vi "Tokenizer Playground.vi"() -> ()   [LabVIEW 2019]
uses:
  Rectangle/Rectangle.lvclass
  ParsePaths/Path.lvclass
  Image/SVGImage.lvclass
  ParseXML/ParseSVG.lvclass
  Image/InitializationInfo.ctl
  ParseXML/ParseSVG.lvclass/ParseSVG.ctl
  Rectangle/InitializeInformation.ctl
panel:
  in  "string":string
  out "Image":refnum<class "SVGImage.lvclass">
  out "Paths":refnum<class "Path.lvclass">[](array[class])
  out "Rectangles":refnum<class "Rectangle.lvclass">[](array[class])
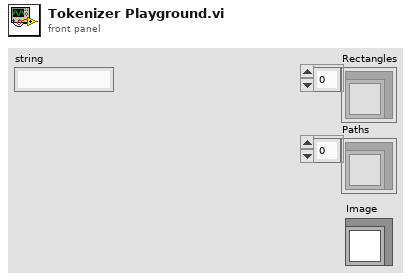
[diagram p1: front panel]
types:
  T1 = typedef "SVGImage.lvclass/InitializationInfo.ctl" = cluster{"X":string, "Y":string, "Width":string, "Height":string, "File Path":string, "ID":string}
  T2 = typedef "ParseSVG.lvclass/Path.ctl" = cluster{"d":string, "style":string, "transform":string, "id":string}
  T3 = typedef "ParseSVG.lvclass/Rect.ctl" = cluster{"style":string, "transform":string, "x":string, "y":string, "width":string, "height":string, "rx":string, "ry":string, "id":string}
  T4 = typedef "Rectangle.lvclass/InitializeInformation.ctl" = cluster{"X":string, "Y":string, "Width":string, "Height":string, "Rx":string, "Ry":string}
  T5 = typedef "ParseSVG.lvclass/Image.ctl" = cluster{"x":string, "y":string, "width":string, "height":string, "xlink:href":string, "id":string}
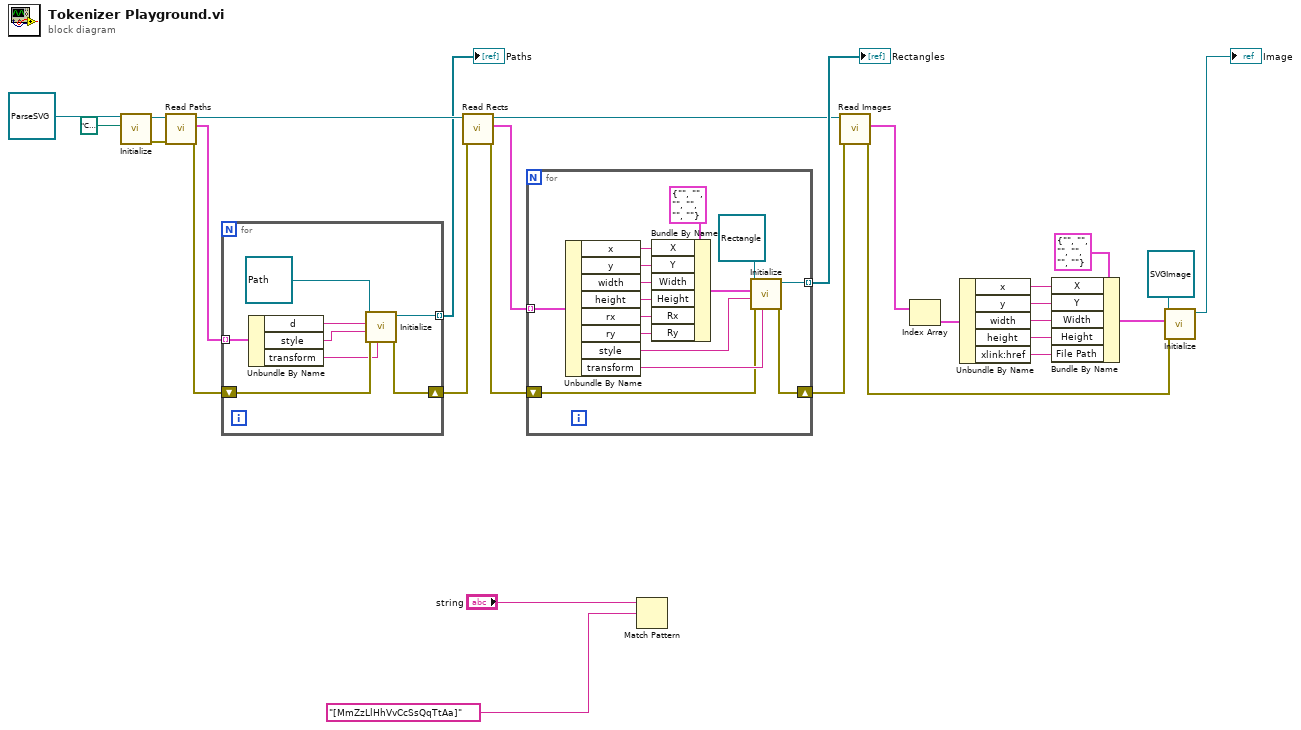
[diagram p0: block diagram]
diagram:
  n1 = call "Initialize.vi"("Path"=path "C:/Users/Albro/Desktop/Rotated Rectangle.svg", "ParseXML in"=refnum<class "ParseSVG.lvclass"> refnum) -> ("error out"=w22:errorcluster, "ParseXML out"=w24:refnum<class "ParseSVG.lvclass">)  [unwired: 8 in]
  n2 = call "Read Paths.vi"("error in (no error)"=w22, "ParseXML in"=w24) -> ("error out"=w27:errorcluster, "Paths"=w28:T2[], "ParseXML out"=w18:refnum<class "ParseSVG.lvclass">)  [unwired: 7 in]
  n3 = for {
    tunnel: w28 -> [w36] mode=indexing
    shift-right: [w31] -> w19
    shift-left: w27 -> [w32]
    tunnel: [w29] -> w17 mode=indexing
    n4 = Unbundle By Name(w36) -> ("d"=w35:string, "style"=w34:string, "transform"=w30:string)
    n5 = call "Initialize.vi"("Path Transform"=w30, "error in (no error)"=w32, "Path Style"=w34, "Path Data"=w35, "Path in"=refnum<class "Path.lvclass"> refnum ("Path.lvclass")) -> ("error out"=w31:errorcluster, "Path out"=w29:refnum<class "Path.lvclass">)  [unwired: 5 in]
  }
  "Paths" <- w17
  n6 = call "Read Rects.vi"("error in (no error)"=w19, "ParseSVG in"=w18) -> ("error out"=w21:errorcluster, "Rects"=w23:T3[], "ParseSVG out"=w16:refnum<class "ParseSVG.lvclass">)  [unwired: 7 in]
  n7 = for {
    tunnel: w23 -> [w51] mode=indexing
    shift-right: [w38] -> w15
    shift-left: w21 -> [w39]
    tunnel: [w37] -> w20 mode=indexing
    n8 = Unbundle By Name(w51) -> ("x"=w49:string, "y"=w48:string, "width"=w47:string, "height"=w46:string, "rx"=w45:string, "ry"=w44:string, "style"=w41:string, "transform"=w40:string)
    n9 = Bundle By Name(cluster=T4 {"X"="", "Y"="", "Width"="", "Height"="", "Rx"="", "Ry"=""} ("rect"), "X"=w49, "Y"=w48, "Width"=w47, "Height"=w46, "Rx"=w45, "Ry"=w44) -> (w42:T4)
    n10 = call "Initialize.vi"("Transform"=w40, "error in (no error)"=w39, "Style"=w41, "rect"=w42, "Rectangle in"=refnum<class "Rectangle.lvclass"> refnum) -> ("error out"=w38:errorcluster, "Rectangle out"=w37:refnum<class "Rectangle.lvclass">)  [unwired: 5 in]
  }
  "Rectangles" <- w20
  n11 = Match Pattern(string="string", regular expression="[MmZzLlHhVvCcSsQqTtAa]") -> ()  [unwired: 1 in, 4 out]
  n12 = call "Read Images.vi"("error in (no error)"=w15, "ParseSVG in"=w16) -> ("error out"=w4:errorcluster, "Images"=w14:T5[])  [unwired: 7 in, 1 out]
  n13 = Index Array(array=w14) -> (element=w13:T5)  [unwired: 1 in]
  n14 = Unbundle By Name(w13) -> ("x"=w11:string, "y"=w10:string, "width"=w9:string, "height"=w8:string, "xlink:href"=w7:string)
  n15 = Bundle By Name(cluster=T1 {"X"="", "Y"="", "Width"="", "Height"="", "File Path"="", "ID"=""} ("Info"), "X"=w11, "Y"=w10, "Width"=w9, "Height"=w8, "File Path"=w7) -> (w6:T1)
  n16 = call "Initialize.vi"("error in (no error)"=w4, "Info"=w6, "Image in"=refnum<class "SVGImage.lvclass"> refnum) -> ("Image out"=→"Image":refnum<class "SVGImage.lvclass">)  [unwired: 7 in, 1 out]
